vi "Phasor Update Gate Step & Number.vi"(8 "Period":dbl[unit], 9 "Value to Update":T1 caption="Parameter to adjust", 10 "# Gates in":dbl, 11 "Gate Step in":dbl[unit]) -> (2 "# Gates out":dbl, 3 "Gate Step out":dbl[unit])   [LabVIEW 2021, in "Phasor.lvlib"]
doc: "Updates gate step number depending on other parameters."
uses:
  Phasor.lvlib
  Phasor Explorer Gate Parameter to Adjust.ctl
  Phasor Explorer.lvlib
panel:
  # "see the AlliGator License on the block diagram (Ctrl+E or Window:Show Block Diagram)"
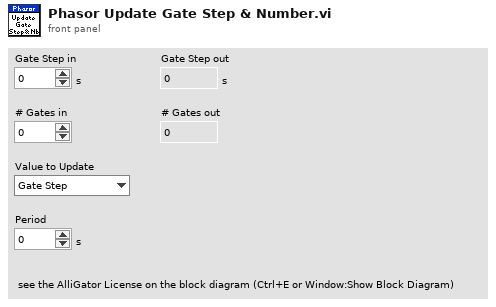
[diagram p1: front panel]
types:
  T1 = typedef "Phasor Explorer.lvlib/Phasor Explorer Gate Parameter to Adjust.ctl" = enum16{"Gate Step", "# Gates"}
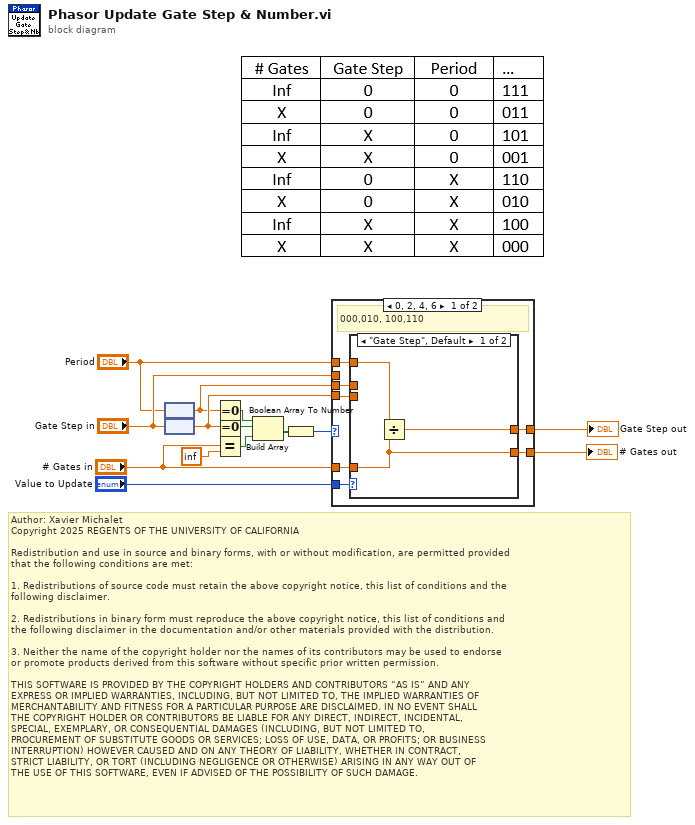
[diagram p0: block diagram]
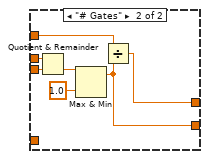
[diagram p2: hidden frame]
diagram:
  # "Author: Xavier Michalet\nCopyright 2025 REGENTS OF THE UNIVERSITY OF CALIFORNIA\n\nRedistribution and use in source and binary forms, with or without modification, are permitted provided\nthat the following conditions are met:\n\n1. Redistributions of source code must retain the above copyright notice, this list of conditions and the\nfollowing disclaimer.\n\n2. Redistributions in binary form must reproduce the above copyright notice, this list of conditions and\nthe following disclaimer in the documentation and/or other materials provided with the distribution.\n\n3. Neither the name of the copyright holder nor the names of its contributors may be used to endorse \nor promote products derived from this software without specific prior written permission.\n\nTHIS SOFTWARE IS PROVIDED BY THE COPYRIGHT HOLDERS AND CONTRIBUTORS “AS IS” AND ANY \nEXPRESS OR IMPLIED WARRANTIES, INCLUDING, BUT NOT LIMITED TO, THE IMPLIED WARRANTIES OF\nMERCHANTABILITY AND FITNESS FOR A PARTICULAR PURPOSE ARE DISCLAIMED. IN NO EVENT SHALL\nTHE COPYRIGHT HOLDER OR CONTRIBUTORS BE LIABLE FOR ANY DIRECT, INDIRECT, INCIDENTAL, \nSPECIAL, EXEMPLARY, OR CONSEQUENTIAL DAMAGES (INCLUDING, BUT NOT LIMITED TO, \nPROCUREMENT OF SUBSTITUTE GOODS OR SERVICES; LOSS OF USE, DATA, OR PROFITS; OR BUSINESS\nINTERRUPTION) HOWEVER CAUSED AND ON ANY THEORY OF LIABILITY, WHETHER IN CONTRACT, \nSTRICT LIABILITY, OR TORT (INCLUDING NEGLIGENCE OR OTHERWISE) ARISING IN ANY WAY OUT OF\nTHE USE OF THIS SOFTWARE, EVEN IF ADVISED OF THE POSSIBILITY OF SUCH DAMAGE."
  n1 = node("Period") -> (w9:dbl)
  n2 = node("Gate Step in") -> (w10:dbl)
  n3 = Equal To 0?(x=w9) -> (x = 0?=w7:bool)
  n4 = Equal To 0?(x=w10) -> (x = 0?=w3:bool)
  n5 = Equal?(x="# Gates in", y=inf) -> (x = y?=w4:bool)
  n6 = Build Array(w7, w3, w4) -> (w5:bool[])
  n7 = Boolean Array To Number(Boolean array=w5) -> (number=w6:u32)
  n8 = case shown="0, 2, 4, 6" w6 {
    tunnel: "Period" -> [w21 _]
    tunnel: "# Gates in" -> [w19 w32]
    tunnel: [w20 w33] -> w11
    tunnel: [w15 w32] -> w12
    tunnel: "Gate Step in" -> [_ w33]
    tunnel: w9 -> [w17 _]
    tunnel: w10 -> [w16 _]
    tunnel: "Value to Update" -> [w18 _]
    frame 0, 2, 4, 6 {
      # "000,010, 100,110"
      n9 = case shown="\"Gate Step\", Default" w18 {
        tunnel: w21 -> [w24 w27]
        tunnel: [w23 w26] -> w20
        tunnel: w19 -> [w22 _]
        tunnel: w17 -> [_ w29]
        tunnel: w16 -> [_ w28]
        tunnel: [w22 w25] -> w15
        frame "Gate Step", Default {
          n10 = Divide(x=w24, y=w22) -> (x/y=w23:dbl[unit])
        }
        frame "# Gates" {
          n11 = Quotient & Remainder(x=w29, y=w28) -> (floor(x/y)=w31:dbl)  [unwired: 1 out]
          n12 = Max & Min(x=w31, y=1.0) -> (max(x,y)=w25:dbl)  [unwired: 1 out]
          n13 = Divide(x=w27, y=w25) -> (x/y=w26:dbl[unit])
        }
      }
    }
    frame 1, Default {
      # "no change"
      # "001, 011, 101, 111"
    }
  }
  "# Gates out" <- w12
  "Gate Step out" <- w11
